vi "GeoData.vi"() -> ()   [LabVIEW 2017] (continued)
Altha\tFL\tCalhoun County\tH1\n32448\t12013\tMarianna\tFL\tCalhoun County\tH1\n32449\t12013\tWewahitchka\tFL\tCalhoun County\tH1\n32442\t12013\tGrand ridge\tFL\tCalhoun County\tH1\n34223\t12015\tEnglewood\tFL\tCharlotte County\tH1\n33950\t12015\tPunta gorda\tFL\tCharlotte County\tH1\n33947\t12015\tRotonda west\tFL\tCharlotte County\tH1\n33953\t12015\tPort charlotte\tFL\tCharlotte County\tH1\n34287\t12015\tNorth port\tFL\tCharlotte County\tH1\n33982\t12015\tPunta gorda\tFL\tCharlotte County\tH1\n34224\t12015\tEnglewood\tFL\tCharlotte County\tH1\n33938\t12015\tMurdock\tFL\tCharlotte County\tH1\n33949\t12015\tPort charlotte\tFL\tCharlotte County\tH1\n33983\t12015\tPunta gorda\tFL\tCharlotte County\tH1\n33952\t12015\tPort charlotte\tFL\tCharlotte County\tH1\n34266\t12015\tArcadia\tFL\tCharlotte County\tH1\n33981\t12015\tPort charlotte\tFL\tCharlotte County\tH1\n33980\t12015\tPunta gorda\tFL\tCharlotte County\tH1\n33946\t12015\tPlacida\tFL\tCharlotte County\tH1\n33954\t12015\tPort charlotte\tFL\tCharlotte County\tH1\n33955\t12015\tPunta gorda\tFL\tCharlotte County\tH1\n33951\t12015\tPunta gorda\tFL\tCharlotte County\tH1\n33917\t12015\tNorth fort myers\tFL\tCharlotte County\tH1\n33948\t12015\tPort charlotte\tFL\tCharlotte County\tH1\n34269\t12015\tArcadia\tFL\tCharlotte County\tH1\n34449\t12017\tInglis\tFL\tCitrus County\tH1\n34428\t12017\tCrystal river\tFL\tCitrus County\tH1\n34601\t12017\tBrooksville\tFL\tCitrus County\tH1\n34460\t12017\tLecanto\tFL\tCitrus County\tH1\n34464\t12017\tBeverly hills\tFL\tCitrus County\tH1\n34452\t12017\tInverness\tFL\tCitrus County\tH1\n34487\t12017\tHomosassa\tFL\tCitrus County\tH1\n34448\t12017\tHomosassa\tFL\tCitrus County\tH1\n34465\t12017\tBeverly hills\tFL\tCitrus County\tH1\n34434\t12017\tDunnellon\tFL\tCitrus County\tH1\n34450\t12017\tInverness\tFL\tCitrus County\tH1\n34436\t12017\tFloral city\tFL\tCitrus County\tH1\n34423\t12017\tCrystal river\tFL\tCitrus County\tH1\n34433\t12017\tDunnellon\tFL\tCitrus County\tH1\n34442\t12017\tHernando\tFL\tCitrus County\tH1\n34453\t12017\tInverness\tFL\tCitrus County\tH1\n34441\t12017\tHernando\tFL\tCitrus County\tH1\n34447\t12017\tHomosassa springs\tFL\tCitrus County\tH1\n34446\t12017\tHomosassa\tFL\tCitrus County\tH1\n34451\t12017\tInverness\tFL\tCitrus County\tH1\n34461\t12017\tLecanto\tFL\tCitrus County\tH1\n34445\t12017\tHolder\tFL\tCitrus County\tH1\n34429\t12017\tCrystal river\tFL\tCitrus County\tH1\n32050\t12019\tMiddleburg\tFL\tClay County\tH1\n32091\t12019\tStarke\tFL\tClay County\tH1\n32234\t12019\tJacksonville\tFL\tClay County\tH1\n32058\t12019\tLawtey\tFL\tClay County\tH1\n32656\t12019\tKeystone heights\tFL\tClay County\tH1\n32140\t12019\tFlorahome\tFL\tClay County\tH1\n32043\t12019\tGreen cove springs\tFL\tClay County\tH1\n32073\t12019\tOrange park\tFL\tClay County\tH1\n32666\t12019\tMelrose\tFL\tClay County\tH1\n32067\t12019\tOrange park\tFL\tClay County\tH1\n32079\t12019\tPenney farms\tFL\tClay County\tH1\n32160\t12019\tLake geneva\tFL\tClay County\tH1\n32003\t12019\tFleming island\tFL\tClay County\tH1\n32068\t12019\tMiddleburg\tFL\tClay County\tH1\n32006\t12019\tFleming island\tFL\tClay County\tH1\n32065\t12019\tOrange park\tFL\tClay County\tH1\n34119\t12021\tNaples\tFL\tCollier County\tH1\n34101\t12021\tNaples\tFL\tCollier County\tH1\n34112\t12021\tNaples\tFL\tCollier County\tH1\n34103\t12021\tNaples\tFL\tCollier County\tH1\n34114\t12021\tNaples\tFL\tCollier County\tH1\n34135\t12021\tBonita springs\tFL\tCollier County\tH1\n34141\t12021\tOchopee\tFL\tCollier County\tH1\n34146\t12021\tMarco island\tFL\tCollier County\tH1\n34110\t12021\tNaples\tFL\tCollier County\tH1\n34120\t12021\tNaples\tFL\tCollier County\tH1\n34134\t12021\tBonita springs\tFL\tCollier County\tH1\n34117\t12021\tNaples\tFL\tCollier County\tH1\n34106\t12021\tNaples\tFL\tCollier County\tH1\n34104\t12021\tNaples\tFL\tCollier County\tH1\n34116\t12021\tNaples\tFL\tCollier County\tH1\n34108\t12021\tNaples\tFL\tCollier County\tH1\n34145\t12021\tMarco island\tFL\tCollier County\tH1\n34140\t12021\tGoodland\tFL\tCollier County\tH1\n34102\t12021\tNaples\tFL\tCollier County\tH1\n34107\t12021\tNaples\tFL\tCollier County\tH1\n34109\t12021\tNaples\tFL\tCollier County\tH1\n34113\t12021\tNaples\tFL\tCollier County\tH1\n34105\t12021\tNaples\tFL\tCollier County\tH1\n34142\t12021\tImmokalee\tFL\tCollier County\tH1\n34139\t12021\tEverglades city\tFL\tCollier County\tH1\n34138\t12021\tChokoloskee\tFL\tCollier County\tH1\n32038\t12023\tFort white\tFL\tColumbia County\tH1\n32025\t12023\tLake city\tFL\tColumbia County\tH1\n32061\t12023\tLulu\tFL\tColumbia County\tH1\n32087\t12023\tSanderson\tFL\tColumbia County\tH1\n32096\t12023\tWhite springs\tFL\tColumbia County\tH1\n32056\t12023\tLake city\tFL\tColumbia County\tH1\n32643\t12023\tHigh springs\tFL\tColumbia County\tH1\n32024\t12023\tLake city\tFL\tColumbia County\tH1\n32055\t12023\tLake city\tFL\tColumbia County\tH1\n32094\t12023\tWellborn\tFL\tColumbia County\tH1\n34268\t12027\tNocatee\tFL\tDeSoto County\tH1\n34267\t12027\tFort ogden\tFL\tDeSoto County\tH1\n34266\t12027\tArcadia\tFL\tDeSoto County\tH1\n33865\t12027\tOna\tFL\tDeSoto County\tH1\n34269\t12027\tArcadia\tFL\tDeSoto County\tH1\n32008\t12029\tBranford\tFL\tDixie County\tH1\n32680\t12029\tOld town\tFL\tDixie County\tH1\n32692\t12029\tSuwannee\tFL\tDixie County\tH1\n32628\t12029\tCross city\tFL\tDixie County\tH1\n32648\t12029\tHorseshoe beach\tFL\tDixie County\tH1\n32359\t12029\tSteinhatchee\tFL\tDixie County\tH1\n32233\t12031\tAtlantic beach\tFL\tDuval County\tH6\n32244\t12031\tJacksonville\tFL\tDuval County\tH6\n32277\t12031\tJacksonville\tFL\tDuval County\tH6\n32209\t12031\tJacksonville\tFL\tDuval County\tH6\n32218\t12031\tJacksonville\tFL\tDuval County\tH6\n32250\t12031\tJacksonville beach\tFL\tDuval County\tH6\n32245\t12031\tJacksonville\tFL\tDuval County\tH6\n32212\t12031\tJacksonville\tFL\tDuval County\tH6\n32228\t12031\tJacksonville\tFL\tDuval County\tH6\n32229\t12031\tJacksonville\tFL\tDuval County\tH6\n32082\t12031\tPonte vedra beach\tFL\tDuval County\tH6\n32081\t12031\tPonte vedra\tFL\tDuval County\tH6\n32224\t12031\tJacksonville\tFL\tDuval County\tH6\n32234\t12031\tJacksonville\tFL\tDuval County\tH6\n32246\t12031\tJacksonville\tFL\tDuval County\tH6\n32214\t12031\tJacksonville\tFL\tDuval County\tH6\n32099\t12031\tJacksonville\tFL\tDuval County\tH6\n32084\t12031\tSaint augustine\tFL\tDuval County\tH6\n32221\t12031\tJacksonville\tFL\tDuval County\tH6\n32223\t12031\tJacksonville\tFL\tDuval County\tH6\n32219\t12031\tJacksonville\tFL\tDuval County\tH6\n32239\t12031\tJacksonville\tFL\tDuval County\tH6\n32227\t12031\tJacksonville\tFL\tDuval County\tH6\n32257\t12031\tJacksonville\tFL\tDuval County\tH6\n32073\t12031\tOrange park\tFL\tDuval County\tH6\n32205\t12031\tJacksonville\tFL\tDuval County\tH6\n32220\t12031\tJacksonville\tFL\tDuval County\tH6\n32226\t12031\tJacksonville\tFL\tDuval County\tH6\n32241\t12031\tJacksonville\tFL\tDuval County\tH6\n32208\t12031\tJacksonville\tFL\tDuval County\tH6\n32202\t12031\tJacksonville\tFL\tDuval County\tH6\n32211\t12031\tJacksonville\tFL\tDuval County\tH6\n32217\t12031\tJacksonville\tFL\tDuval County\tH6\n32222\t12031\tJacksonville\tFL\tDuval County\tH6\n32240\t12031\tJacksonville beach\tFL\tDuval County\tH6\n32254\t12031\tJacksonville\tFL\tDuval County\tH6\n32259\t12031\tSaint johns\tFL\tDuval County\tH6\n32235\t12031\tJacksonville\tFL\tDuval County\tH6\n32247\t12031\tJacksonville\tFL\tDuval County\tH6\n32206\t12031\tJacksonville\tFL\tDuval County\tH6\n32210\t12031\tJacksonville\tFL\tDuval County\tH6\n32216\t12031\tJacksonville\tFL\tDuval County\tH6\n32236\t12031\tJacksonville\tFL\tDuval County\tH6\n32256\t12031\tJacksonville\tFL\tDuval County\tH6\n32258\t12031\tJacksonville\tFL\tDuval County\tH6\n32255\t12031\tJacksonville\tFL\tDuval County\tH6\n32203\t12031\tJacksonville\tFL\tDuval County\tH6\n32204\t12031\tJacksonville\tFL\tDuval County\tH6\n32207\t12031\tJacksonville\tFL\tDuval County\tH6\n32225\t12031\tJacksonville\tFL\tDuval County\tH6\n32266\t12031\tNeptune beach\tFL\tDuval County\tH6\n32238\t12031\tJacksonville\tFL\tDuval County\tH6\n32506\t12033\tPensacola\tFL\tEscambia County\tH1\n32535\t12033\tCentury\tFL\tEscambia County\tH1\n32503\t12033\tPensacola\tFL\tEscambia County\tH1\n32520\t12033\tPensacola\tFL\tEscambia County\tH1\n32507\t12033\tPensacola\tFL\tEscambia County\tH1\n32524\t12033\tPensacola\tFL\tEscambia County\tH1\n32505\t12033\tPensacola\tFL\tEscambia County\tH1\n32568\t12033\tMc david\tFL\tEscambia County\tH1\n32511\t12033\tPensacola\tFL\tEscambia County\tH1\n32502\t12033\tPensacola\tFL\tEscambia County\tH1\n32534\t12033\tPensacola\tFL\tEscambia County\tH1\n32523\t12033\tPensacola\tFL\tEscambia County\tH1\n32577\t12033\tMolino\tFL\tEscambia County\tH1\n32560\t12033\tGonzalez\tFL\tEscambia County\tH1\n32509\t12033\tPensacola\tFL\tEscambia County\tH1\n32512\t12033\tPensacola\tFL\tEscambia County\tH1\n32504\t12033\tPensacola\tFL\tEscambia County\tH1\n32514\t12033\tPensacola\tFL\tEscambia County\tH1\n32526\t12033\tPensacola\tFL\tEscambia County\tH1\n32561\t12033\tGulf breeze\tFL\tEscambia County\tH1\n32513\t12033\tPensacola\tFL\tEscambia County\tH1\n32508\t12033\tPensacola\tFL\tEscambia County\tH1\n32516\t12033\tPensacola\tFL\tEscambia County\tH1\n32501\t12033\tPensacola\tFL\tEscambia County\tH1\n32522\t12033\tPensacola\tFL\tEscambia County\tH1\n32591\t12033\tPensacola\tFL\tEscambia County\tH1\n32533\t12033\tCantonment\tFL\tEscambia County\tH1\n32559\t12033\tPensacola\tFL\tEscambia County\tH1\n32145\t12035\tHastings\tFL\tFlagler County\tH1\n32143\t12035\tPalm coast\tFL\tFlagler County\tH1\n32110\t12035\tBunnell\tFL\tFlagler County\tH1\n32086\t12035\tSaint augustine\tFL\tFlagler County\tH1\n32136\t12035\tFlagler beach\tFL\tFlagler County\tH1\n32174\t12035\tOrmond beach\tFL\tFlagler County\tH1\n32164\t12035\tPalm coast\tFL\tFlagler County\tH1\n32135\t12035\tPalm coast\tFL\tFlagler County\tH1\n32080\t12035\tSaint augustine\tFL\tFlagler County\tH1\n32137\t12035\tPalm coast\tFL\tFlagler County\tH1\n32320\t12037\tApalachicola\tFL\tFranklin County\tH1\n32322\t12037\tCarrabelle\tFL\tFranklin County\tH1\n32358\t12037\tSopchoppy\tFL\tFranklin County\tH1\n32321\t12037\tBristol\tFL\tFranklin County\tH1\n32346\t12037\tPanacea\tFL\tFranklin County\tH1\n32328\t12037\tEastpoint\tFL\tFranklin County\tH1\n32324\t12039\tChattahoochee\tFL\tGadsden County\tH1\n32352\t12039\tQuincy\tFL\tGadsden County\tH1\n32332\t12039\tGretna\tFL\tGadsden County\tH1\n32343\t12039\tMidway\tFL\tGadsden County\tH1\n32330\t12039\tGreensboro\tFL\tGadsden County\tH1\n32351\t12039\tQuincy\tFL\tGadsden County\tH1\n32333\t12039\tHavana\tFL\tGadsden County\tH1\n32008\t12041\tBranford\tFL\tGilchrist County\tH1\n32669\t12041\tNewberry\tFL\tGilchrist County\tH1\n32619\t12041\tBell\tFL\tGilchrist County\tH1\n32693\t12041\tTrenton\tFL\tGilchrist County\tH1\n32643\t12041\tHigh springs\tFL\tGilchrist County\tH1\n33944\t12043\tPalmdale\tFL\tGlades County\tH1\n33471\t12043\tMoore haven\tFL\tGlades County\tH1\n34974\t12043\tOkeechobee\tFL\tGlades County\tH1\n33935\t12043\tLabelle\tFL\tGlades County\tH1\n33960\t12043\tVenus\tFL\tGlades County\tH1\n32456\t12045\tPort saint joe\tFL\tGulf County\tH1\n32465\t12045\tWewahitchka\tFL\tGulf County\tH1\n32052\t12047\tJasper\tFL\tHamilton County\tH1\n32053\t12047\tJennings\tFL\tHamilton County\tH1\n32096\t12047\tWhite springs\tFL\tHamilton County\tH1\n33841\t12049\tFort meade\tFL\tHardee County\tH1\n33873\t12049\tWauchula\tFL\tHardee County\tH1\n33890\t12049\tZolfo springs\tFL\tHardee County\tH1\n33834\t12049\tBowling green\tFL\tHardee County\tH1\n33865\t12049\tOna\tFL\tHardee County\tH1\n33975\t12051\tLabelle\tFL\tHendry County\tH1\n33471\t12051\tMoore haven\tFL\tHendry County\tH1\n33935\t12051\tLabelle\tFL\tHendry County\tH1\n33440\t12051\tClewiston\tFL\tHendry County\tH1\n33930\t12051\tFelda\tFL\tHendry County\tH1\n33936\t12051\tLehigh acres\tFL\tHendry County\tH1\n34142\t12051\tImmokalee\tFL\tHendry County\tH1\n34601\t12053\tBrooksville\tFL\tHernando County\tH1\n33523\t12053\tDade city\tFL\tHernando County\tH1\n33597\t12053\tWebster\tFL\tHernando County\tH1\n34613\t12053\tBrooksville\tFL\tHernando County\tH1\n34606\t12053\tSpring hill\tFL\tHernando County\tH1\n34608\t12053\tSpring hill\tFL\tHernando County\tH1\n34609\t12053\tSpring hill\tFL\tHernando County\tH1\n34607\t12053\tSpring hill\tFL\tHernando County\tH1\n34636\t12053\tIstachatta\tFL\tHernando County\tH1\n34604\t12053\tBrooksville\tFL\tHernando County\tH1\n34603\t12053\tBrooksville\tFL\tHernando County\tH1\n34602\t12053\tBrooksville\tFL\tHernando County\tH1\n34661\t12053\tNobleton\tFL\tHernando County\tH1\n34605\t12053\tBrooksville\tFL\tHernando County\tH1\n34614\t12053\tBrooksville\tFL\tHernando County\tH1\n34611\t12053\tSpring hill\tFL\tHernando County\tH1\n33843\t12055\tFrostproof\tFL\tHighlands County\tH1\n33875\t12055\tSebring\tFL\tHighlands County\tH1\n33862\t12055\tLake placid\tFL\tHighlands County\tH1\n33825\t12055\tAvon park\tFL\tHighlands County\tH1\n33876\t12055\tSebring\tFL\tHighlands County\tH1\n33871\t12055\tSebring\tFL\tHighlands County\tH1\n34974\t12055\tOkeechobee\tFL\tHighlands County\tH1\n33852\t12055\tLake placid\tFL\tHighlands County\tH1\n33870\t12055\tSebring\tFL\tHighlands County\tH1\n34266\t12055\tArcadia\tFL\tHighlands County\tH1\n33857\t12055\tLorida\tFL\tHighlands County\tH1\n33872\t12055\tSebring\tFL\tHighlands County\tH1\n33960\t12055\tVenus\tFL\tHighlands County\tH1\n33511\t12057\tBrandon\tFL\tHillsborough County\tH1\n33570\t12057\tRuskin\tFL\tHillsborough County\tH1\n33573\t12057\tSun city center\tFL\tHillsborough County\tH1\n33564\t12057\tPlant city\tFL\tHillsborough County\tH1\n33547\t12057\tLithia\tFL\tHillsborough County\tH1\n33583\t12057\tSeffner\tFL\tHillsborough County\tH1\n33614\t12057\tTampa\tFL\tHillsborough County\tH1\n33610\t12057\tTampa\tFL\tHillsborough County\tH1\n33616\t12057\tTampa\tFL\tHillsborough County\tH1\n33568\t12057\tRiverview\tFL\tHillsborough County\tH1\n33680\t12057\tTampa\tFL\tHillsborough County\tH1\n33694\t12057\tTampa\tFL\tHillsborough County\tH1\n33679\t12057\tTampa\tFL\tHillsborough County\tH1\n33565\t12057\tPlant city\tFL\tHillsborough County\tH1\n33544\t12057\tWesley chapel\tFL\tHillsborough County\tH1\n33605\t12057\tTampa\tFL\tHillsborough County\tH1\n33548\t12057\tLutz\tFL\tHillsborough County\tH1\n33617\t12057\tTampa\tFL\tHillsborough County\tH1\n33625\t12057\tTampa\tFL\tHillsborough County\tH1\n33615\t12057\tTampa\tFL\tHillsborough County\tH1\n33688\t12057\tTampa\tFL\tHillsborough County\tH1\n33558\t12057\tLutz\tFL\tHillsborough County\tH1\n33569\t12057\tRiverview\tFL\tHillsborough County\tH1\n33595\t12057\tValrico\tFL\tHillsborough County\tH1\n33611\t12057\tTampa\tFL\tHillsborough County\tH1\n33684\t12057\tTampa\tFL\tHillsborough County\tH1\n33620\t12057\tTampa\tFL\tHillsborough County\tH1\n33672\t12057\tTampa\tFL\tHillsborough County\tH1\n33646\t12057\tTampa\tFL\tHillsborough County\tH1\n33673\t12057\tTampa\tFL\tHillsborough County\tH1\n33630\t12057\tTampa\tFL\tHillsborough County\tH1\n33563\t12057\tPlant city\tFL\tHillsborough County\tH1\n33578\t12057\tRiverview\tFL\tHillsborough County\tH1\n33584\t12057\tSeffner\tFL\tHillsborough County\tH1\n33592\t12057\tThonotosassa\tFL\tHillsborough County\tH1\n33594\t12057\tValrico\tFL\tHillsborough County\tH1\n33623\t12057\tTampa\tFL\tHillsborough County\tH1\n33689\t12057\tTampa\tFL\tHillsborough County\tH1\n33674\t12057\tTampa\tFL\tHillsborough County\tH1\n33586\t12057\tSun city\tFL\tHillsborough County\tH1\n33549\t12057\tLutz\tFL\tHillsborough County\tH1\n33566\t12057\tPlant city\tFL\tHillsborough County\tH1\n33527\t12057\tDover\tFL\tHillsborough County\tH1\n33604\t12057\tTampa\tFL\tHillsborough County\tH1\n33598\t12057\tWimauma\tFL\tHillsborough County\tH1\n33624\t12057\tTampa\tFL\tHillsborough County\tH1\n33635\t12057\tTampa\tFL\tHillsborough County\tH1\n33687\t12057\tTampa\tFL\tHillsborough County\tH1\n33681\t12057\tTampa\tFL\tHillsborough County\tH1\n33559\t12057\tLutz\tFL\tHillsborough County\tH1\n33579\t12057\tRiverview\tFL\tHillsborough County\tH1\n33601\t12057\tTampa\tFL\tHillsborough County\tH1\n33602\t12057\tTampa\tFL\tHillsborough County\tH1\n33572\t12057\tApollo beach\tFL\tHillsborough County\tH1\n33550\t12057\tMango\tFL\tHillsborough County\tH1\n33596\t12057\tValrico\tFL\tHillsborough County\tH1\n33647\t12057\tTampa\tFL\tHillsborough County\tH1\n33626\t12057\tTampa\tFL\tHillsborough County\tH1\n33622\t12057\tTampa\tFL\tHillsborough County\tH1\n33609\t12057\tTampa\tFL\tHillsborough County\tH1\n33860\t12057\tMulberry\tFL\tHillsborough County\tH1\n33810\t12057\tLakeland\tFL\tHillsborough County\tH1\n33509\t12057\tBrandon\tFL\tHillsborough County\tH1\n33530\t12057\tDurant\tFL\tHillsborough County\tH1\n33675\t12057\tTampa\tFL\tHillsborough County\tH1\n33540\t12057\tZephyrhills\tFL\tHillsborough County\tH1\n33618\t12057\tTampa\tFL\tHillsborough County\tH1\n33629\t12057\tTampa\tFL\tHillsborough County\tH1\n33682\t12057\tTampa\tFL\tHillsborough County\tH1\n33621\t12057\tTampa\tFL\tHillsborough County\tH1\n33677\t12057\tTampa\tFL\tHillsborough County\tH1\n33571\t12057\tSun city center\tFL\tHillsborough County\tH1\n33503\t12057\tBalm\tFL\tHillsborough County\tH1\n33510\t12057\tBrandon\tFL\tHillsborough County\tH1\n33556\t12057\tOdessa\tFL\tHillsborough County\tH1\n33567\t12057\tPlant city\tFL\tHillsborough County\tH1\n33534\t12057\tGibsonton\tFL\tHillsborough County\tH1\n33606\t12057\tTampa\tFL\tHillsborough County\tH1\n33603\t12057\tTampa\tFL\tHillsborough County\tH1\n33613\t12057\tTampa\tFL\tHillsborough County\tH1\n33619\t12057\tTampa\tFL\tHillsborough County\tH1\n33634\t12057\tTampa\tFL\tHillsborough County\tH1\n33607\t12057\tTampa\tFL\tHillsborough County\tH1\n33612\t12057\tTampa\tFL\tHillsborough County\tH1\n33637\t12057\tTampa\tFL\tHillsborough County\tH1\n33685\t12057\tTampa\tFL\tHillsborough County\tH1\n33508\t12057\tBrandon\tFL\tHillsborough County\tH1\n33587\t12057\tSydney\tFL\tHillsborough County\tH1\n32455\t12059\tPonce de leon\tFL\tHolmes County\tH1\n32464\t12059\tWestville\tFL\tHolmes County\tH1\n32425\t12059\tBonifay\tFL\tHolmes County\tH1\n32433\t12059\tDefuniak springs\tFL\tHolmes County\tH1\n32440\t12059\tGraceville\tFL\tHolmes County\tH1\n32452\t12059\tNoma\tFL\tHolmes County\tH1\n32963\t12061\tVero beach\tFL\tIndian River County\tH1\n32965\t12061\tVero beach\tFL\tIndian River County\tH1\n32958\t12061\tSebastian\tFL\tIndian River County\tH1\n32966\t12061\tVero beach\tFL\tIndian River County\tH1\n32969\t12061\tVero beach\tFL\tIndian River County\tH1\n32960\t12061\tVero beach\tFL\tIndian River County\tH1\n32964\t12061\tVero beach\tFL\tIndian River County\tH1\n32957\t12061\tRoseland\tFL\tIndian River County\tH1\n32968\t12061\tVero beach\tFL\tIndian River County\tH1\n32961\t12061\tVero beach\tFL\tIndian River County\tH1\n32978\t12061\tSebastian\tFL\tIndian River County\tH1\n32948\t12061\tFellsmere\tFL\tIndian River County\tH1\n32967\t12061\tVero beach\tFL\tIndian River County\tH1\n32971\t12061\tWinter beach\tFL\tIndian River County\tH1\n32962\t12061\tVero beach\tFL\tIndian River County\tH1\n32970\t12061\tWabasso\tFL\tIndian River County\tH1\n32443\t12063\tGreenwood\tFL\tJackson County\tH1\n32428\t12063\tChipley\tFL\tJackson County\tH1\n32420\t12063\tAlford\tFL\tJackson County\tH1\n32438\t12063\tFountain\tFL\tJackson County\tH1\n32431\t12063\tCottondale\tFL\tJackson County\tH1\n32432\t12063\tCypress\tFL\tJackson County\tH1\n32423\t12063\tBascom\tFL\tJackson County\tH1\n32426\t12063\tCampbellton\tFL\tJackson County\tH1\n32445\t12063\tMalone\tFL\tJackson County\tH1\n32447\t12063\tMarianna\tFL\tJackson County\tH1\n32460\t12063\tSneads\tFL\tJackson County\tH1\n32440\t12063\tGraceville\tFL\tJackson County\tH1\n32446\t12063\tMarianna\tFL\tJackson County\tH1\n32448\t12063\tMarianna\tFL\tJackson County\tH1\n32442\t12063\tGrand ridge\tFL\tJackson County\tH1\n32309\t12065\tTallahassee\tFL\tJefferson County\tH1\n32331\t12065\tGreenville\tFL\tJefferson County\tH1\n32336\t12065\tLamont\tFL\tJefferson County\tH1\n32345\t12065\tMonticello\tFL\tJefferson County\tH1\n32361\t12065\tWacissa\tFL\tJefferson County\tH1\n32344\t12065\tMonticello\tFL\tJefferson County\tH1\n32337\t12065\tLloyd\tFL\tJefferson County\tH1\n32008\t12067\tBranford\tFL\tLafayette County\tH1\n32066\t12067\tMayo\tFL\tLafayette County\tH1\n32195\t12069\tWeirsdale\tFL\tLake County\tH1\n34731\t12069\tFruitland park\tFL\tLake County\tH1\n34729\t12069\tFerndale\tFL\tLake County\tH1\n32776\t12069\tSorrento\tFL\tLake County\tH1\n32784\t12069\tUmatilla\tFL\tLake County\tH1\n34797\t12069\tYalaha\tFL\tLake County\tH1\n32134\t12069\tFort mc coy\tFL\tLake County\tH1\n32163\t12069\tThe villages\tFL\tLake County\tH1\n32756\t12069\tMount dora\tFL\tLake County\tH1\n32767\t12069\tPaisley\tFL\tLake County\tH1\n34711\t12069\tClermont\tFL\tLake County\tH1\n34715\t12069\tClermont\tFL\tLake County\tH1\n34713\t12069\tClermont\tFL\tLake County\tH1\n32158\t12069\tLady lake\tFL\tLake County\tH1\n34756\t12069\tMontverde\tFL\tLake County\tH1\n32727\t12069\tEustis\tFL\tLake County\tH1\n32159\t12069\tLady lake\tFL\tLake County\tH1\n32757\t12069\tMount dora\tFL\tLake County\tH1\n34714\t12069\tClermont\tFL\tLake County\tH1\n34789\t12069\tLeesburg\tFL\tLake County\tH1\n34755\t12069\tMinneola\tFL\tLake County\tH1\n32102\t12069\tAstor\tFL\tLake County\tH1\n34712\t12069\tClermont\tFL\tLake County\tH1\n32702\t12069\tAltoona\tFL\tLake County\tH1\n32736\t12069\tEustis\tFL\tLake County\tH1\n34736\t12069\tGroveland\tFL\tLake County\tH1\n34748\t12069\tLeesburg\tFL\tLake County\tH1\n34762\t12069\tOkahumpka\tFL\tLake County\tH1\n34787\t12069\tWinter garden\tFL\tLake County\tH1\n34753\t12069\tMascotte\tFL\tLake County\tH1\n34705\t12069\tAstatula\tFL\tLake County\tH1\n34749\t12069\tLeesburg\tFL\tLake County\tH1\n32162\t12069\tThe villages\tFL\tLake County\tH1\n32720\t12069\tDeland\tFL\tLake County\tH1\n32726\t12069\tEustis\tFL\tLake County\tH1\n32778\t12069\tTavares\tFL\tLake County\tH1\n32735\t12069\tGrand island\tFL\tLake County\tH1\n34788\t12069\tLeesburg\tFL\tLake County\tH1\n34737\t12069\tHowey in the hills\tFL\tLake County\tH1\n33907\t12071\tFort myers\tFL\tLee County\tH1\n33908\t12071\tFort myers\tFL\tLee County\tH1\n33904\t12071\tCape coral\tFL\tLee County\tH1\n33916\t12071\tFort myers\tFL\tLee County\tH1\n33976\t12071\tLehigh acres\tFL\tLee County\tH1\n33922\t12071\tBokeelia\tFL\tLee County\tH1\n34119\t12071\tNaples\tFL\tLee County\tH1\n33991\t12071\tCape coral\tFL\tLee County\tH1\n33901\t12071\tFort myers\tFL\tLee County\tH1\n33971\t12071\tLehigh acres\tFL\tLee County\tH1\n33972\t12071\tLehigh acres\tFL\tLee County\tH1\n33956\t12071\tSaint james city\tFL\tLee County\tH1\n33990\t12071\tCape coral\tFL\tLee County\tH1\n34133\t12071\tBonita springs\tFL\tLee County\tH1\n33913\t12071\tFort myers\tFL\tLee County\tH1\n33914\t12071\tCape coral\tFL\tLee County\tH1\n33973\t12071\tLehigh acres\tFL\tLee County\tH1\n33919\t12071\tFort myers\tFL\tLee County\tH1\n33906\t12071\tFort myers\tFL\tLee County\tH1\n34135\t12071\tBonita springs\tFL\tLee County\tH1\n33903\t12071\tNorth fort myers\tFL\tLee County\tH1\n33902\t12071\tFort myers\tFL\tLee County\tH1\n33970\t12071\tLehigh acres\tFL\tLee County\tH1\n33965\t12071\tFort myers\tFL\tLee County\tH1\n33928\t12071\tEstero\tFL\tLee County\tH1\n33905\t12071\tFort myers\tFL\tLee County\tH1\n33915\t12071\tCape coral\tFL\tLee County\tH1\n34110\t12071\tNaples\tFL\tLee County\tH1\n34134\t12071\tBonita springs\tFL\tLee County\tH1\n33994\t12071\tFort myers\tFL\tLee County\tH1\n33924\t12071\tCaptiva\tFL\tLee County\tH1\n33912\t12071\tFort myers\tFL\tLee County\tH1\n33957\t12071\tSanibel\tFL\tLee County\tH1\n33974\t12071\tLehigh acres\tFL\tLee County\tH1\n33993\t12071\tCape coral\tFL\tLee County\tH1\n33918\t12071\tNorth fort myers\tFL\tLee County\tH1\n33910\t12071\tCape coral\tFL\tLee County\tH1\n33945\t12071\tPineland\tFL\tLee County\tH1\n33921\t12071\tBoca grande\tFL\tLee County\tH1\n33920\t12071\tAlva\tFL\tLee County\tH1\n33967\t12071\tFort myers\tFL\tLee County\tH1\n33966\t12071\tFort myers\tFL\tLee County\tH1\n33955\t12071\tPunta gorda\tFL\tLee County\tH1\n34136\t12071\tBonita springs\tFL\tLee County\tH1\n33917\t12071\tNorth fort myers\tFL\tLee County\tH1\n33936\t12071\tLehigh acres\tFL\tLee County\tH1\n33909\t12071\tCape coral\tFL\tLee County\tH1\n33931\t12071\tFort myers beach\tFL\tLee County\tH1\n33932\t12071\tFort myers beach\tFL\tLee County\tH1\n33929\t12071\tEstero\tFL\tLee County\tH1\n33911\t12071\tFort myers\tFL\tLee County\tH1\n32305\t12073\tTallahassee\tFL\tLeon County\tH1\n32315\t12073\tTallahassee\tFL\tLeon County\tH1\n32399\t12073\tTallahassee\tFL\tLeon County\tH1\n32314\t12073\tTallahassee\tFL\tLeon County\tH1\n32302\t12073\tTallahassee\tFL\tLeon County\tH1\n32313\t12073\tTallahassee\tFL\tLeon County\tH1\n32304\t12073\tTallahassee\tFL\tLeon County\tH1\n32309\t12073\tTallahassee\tFL\tLeon County\tH1\n32327\t12073\tCrawfordville\tFL\tLeon County\tH1\n32311\t12073\tTallahassee\tFL\tLeon County\tH1\n32318\t12073\tTallahassee\tFL\tLeon County\tH1\n32303\t12073\tTallahassee\tFL\tLeon County\tH1\n32308\t12073\tTallahassee\tFL\tLeon County\tH1\n32310\t12073\tTallahassee\tFL\tLeon County\tH1\n32312\t12073\tTallahassee\tFL\tLeon County\tH1\n32362\t12073\tWoodville\tFL\tLeon County\tH1\n32301\t12073\tTallahassee\tFL\tLeon County\tH1\n32317\t12073\tTallahassee\tFL\tLeon County\tH1\n32306\t12073\tTallahassee\tFL\tLeon County\tH1\n32307\t12073\tTallahassee\tFL\tLeon County\tH1\n32395\t12073\tTallahassee\tFL\tLeon County\tH1\n32316\t12073\tTallahassee\tFL\tLeon County\tH1\n34449\t12075\tInglis\tFL\tLevy County\tH1\n32626\t12075\tChiefland\tFL\tLevy County\tH1\n32621\t12075\tBronson\tFL\tLevy County\tH1\n32669\t12075\tNewberry\tFL\tLevy County\tH1\n32693\t12075\tTrenton\tFL\tLevy County\tH1\n32683\t12075\tOtter creek\tFL\tLevy County\tH1\n32618\t12075\tArcher\tFL\tLevy County\tH1\n32696\t12075\tWilliston\tFL\tLevy County\tH1\n32639\t12075\tGulf hammock\tFL\tLevy County\tH1\n32625\t12075\tCedar key\tFL\tLevy County\tH1\n34498\t12075\tYankeetown\tFL\tLevy County\tH1\n32668\t12075\tMorriston\tFL\tLevy County\tH1\n34431\t12075\tDunnellon\tFL\tLevy County\tH1\n32644\t12075\tChiefland\tFL\tLevy County\tH1\n32334\t12077\tHosford\tFL\tLiberty County\tH1\n32321\t12077\tBristol\tFL\tLiberty County\tH1\n32351\t12077\tQuincy\tFL\tLiberty County\tH1\n32360\t12077\tTelogia\tFL\tLiberty County\tH1\n32350\t12079\tPinetta\tFL\tMadison County\tH1\n32331\t12079\tGreenville\tFL\tMadison County\tH1\n32336\t12079\tLamont\tFL\tMadison County\tH1\n32059\t12079\tLee\tFL\tMadison County\tH1\n32340\t12079\tMadison\tFL\tMadison County\tH1\n34208\t12081\tBradenton\tFL\tManatee County\tH1\n34264\t12081\tOneco\tFL\tManatee County\tH1\n34270\t12081\tTallevast\tFL\tManatee County\tH1\n34206\t12081\tBradenton\tFL\tManatee County\tH1\n34221\t12081\tPalmetto\tFL\tManatee County\tH1\n34209\t12081\tBradenton\tFL\tManatee County\tH1\n34217\t12081\tBradenton beach\tFL\tManatee County\tH1\n34222\t12081\tEllenton\tFL\tManatee County\tH1\n34251\t12081\tMyakka city\tFL\tManatee County\tH1\n34243\t12081\tSarasota\tFL\tManatee County\tH1\n34205\t12081\tBradenton\tFL\tManatee County\tH1\n34280\t12081\tBradenton\tFL\tManatee County\tH1\n34216\t12081\tAnna maria\tFL\tManatee County\tH1\n34282\t12081\tBradenton\tFL\tManatee County\tH1\n34228\t12081\tLongboat key\tFL\tManatee County\tH1\n34202\t12081\tBradenton\tFL\tManatee County\tH1\n34211\t12081\tBradenton\tFL\tManatee County\tH1\n34240\t12081\tSarasota\tFL\tManatee County\tH1\n34212\t12081\tBradenton\tFL\tManatee County\tH1\n34201\t12081\tBradenton\tFL\tManatee County\tH1\n33598\t12081\tWimauma\tFL\tManatee County\tH1\n34266\t12081\tArcadia\tFL\tManatee County\tH1\n34220\t12081\tPalmetto\tFL\tManatee County\tH1\n33834\t12081\tBowling green\tFL\tManatee County\tH1\n34210\t12081\tBradenton\tFL\tManatee County\tH1\n34219\t12081\tParrish\tFL\tManatee County\tH1\n34203\t12081\tBradenton\tFL\tManatee County\tH1\n34204\t12081\tBradenton\tFL\tManatee County\tH1\n34260\t12081\tSarasota\tFL\tManatee County\tH1\n34250\t12081\tTerra ceia\tFL\tManatee County\tH1\n34207\t12081\tBradenton\tFL\tManatee County\tH1\n34215\t12081\tCortez\tFL\tManatee County\tH1\n32195\t12083\tWeirsdale\tFL\tMarion County\tH1\n32182\t12083\tOrange springs\tFL\tMarion County\tH1\n34471\t12083\tOcala\tFL\tMarion County\tH1\n34480\t12083\tOcala\tFL\tMarion County\tH1\n34482\t12083\tOcala\tFL\tMarion County\tH1\n32784\t12083\tUmatilla\tFL\tMarion County\tH1\n32664\t12083\tMc intosh\tFL\tMarion County\tH1\n34430\t12083\tDunnellon\tFL\tMarion County\tH1\n32663\t12083\tLowell\tFL\tMarion County\tH1\n32111\t12083\tCandler\tFL\tMarion County\tH1\n34491\t12083\tSummerfield\tFL\tMarion County\tH1\n34475\t12083\tOcala\tFL\tMarion County\tH1\n34481\t12083\tOcala\tFL\tMarion County\tH1\n32134\t12083\tFort mc coy\tFL\tMarion County\tH1\n32113\t12083\tCitra\tFL\tMarion County\tH1\n32667\t12083\tMicanopy\tFL\tMarion County\tH1\n34473\t12083\tOcala\tFL\tMarion County\tH1\n34474\t12083\tOcala\tFL\tMarion County\tH1\n32634\t12083\tFairfield\tFL\tMarion County\tH1\n34472\t12083\tOcala\tFL\tMarion County\tH1\n34476\t12083\tOcala\tFL\tMarion County\tH1\n32192\t12083\tSparr\tFL\tMarion County\tH1\n32681\t12083\tOrange lake\tFL\tMarion County\tH1\n32133\t12083\tEastlake weir\tFL\tMarion County\tH1\n32696\t12083\tWilliston\tFL\tMarion County\tH1\n34420\t12083\tBelleview\tFL\tMarion County\tH1\n34477\t12083\tOcala\tFL\tMarion County\tH1\n34492\t12083\tSummerfield\tFL\tMarion County\tH1\n34483\t12083\tOcala\tFL\tMarion County\tH1\n32686\t12083\tReddick\tFL\tMarion County\tH1\n34470\t12083\tOcala\tFL\tMarion County\tH1\n32702\t12083\tAltoona\tFL\tMarion County\tH1\n32617\t12083\tAnthony\tFL\tMarion County\tH1\n32668\t12083\tMorriston\tFL\tMarion County\tH1\n34431\t12083\tDunnellon\tFL\tMarion County\tH1\n34432\t12083\tDunnellon\tFL\tMarion County\tH1\n34484\t12083\tOxford\tFL\tMarion County\tH1\n34488\t12083\tSilver springs\tFL\tMarion County\tH1\n34478\t12083\tOcala\tFL\tMarion County\tH1\n34479\t12083\tOcala\tFL\tMarion County\tH1\n32162\t12083\tThe villages\tFL\tMarion County\tH1\n32179\t12083\tOcklawaha\tFL\tMarion County\tH1\n34489\t12083\tSilver springs\tFL\tMarion County\tH1\n33478\t12085\tJupiter\tFL\tMartin County\tH1\n34994\t12085\tStuart\tFL\tMartin County\tH1\n34956\t12085\tIndiantown\tFL\tMartin County\tH1\n34995\t12085\tStuart\tFL\tMartin County\tH1\n34974\t12085\tOkeechobee\tFL\tMartin County\tH1\n34957\t12085\tJensen beach\tFL\tMartin County\tH1\n34996\t12085\tStuart\tFL\tMartin County\tH1\n34958\t12085\tJensen beach\tFL\tMartin County\tH1\n34992\t12085\tPort salerno\tFL\tMartin County\tH1\n33438\t12085\tCanal point\tFL\tMartin County\tH1\n33458\t12085\tJupiter\tFL\tMartin County\tH1\n33475\t12085\tHobe sound\tFL\tMartin County\tH1\n33455\t12085\tHobe sound\tFL\tMartin County\tH1\n34990\t12085\tPalm city\tFL\tMartin County\tH1\n34991\t12085\tPalm city\tFL\tMartin County\tH1\n33469\t12085\tJupiter\tFL\tMartin County\tH1\n34997\t12085\tStuart\tFL\tMartin County\tH1\n33015\t12086\tHialeah\tFL\tMiami-Dade County\tH1\n33137\t12086\tMiami\tFL\tMiami-Dade County\tH1\n33176\t12086\tMiami\tFL\tMiami-Dade County\tH1\n33166\t12086\tMiami\tFL\tMiami-Dade County\tH1\n33283\t12086\tMiami\tFL\tMiami-Dade County\tH1\n33030\t12086\tHomestead\tFL\tMiami-Dade County\tH1\n33114\t12086\tCoral gables\tFL\tMiami-Dade County\tH1\n33116\t12086\tMiami\tFL\tMiami-Dade County\tH1\n33002\t12086\tHialeah\tFL\tMiami-Dade County\tH1\n33192\t12086\tMiami\tFL\tMiami-Dade County\tH1\n33199\t12086\tMiami\tFL\tMiami-Dade County\tH1\n33129\t12086\tMiami\tFL\tMiami-Dade County\tH1\n33109\t12086\tMiami beach\tFL\tMiami-Dade County\tH1\n33127\t12086\tMiami\tFL\tMiami-Dade County\tH1\n33145\t12086\tMiami\tFL\tMiami-Dade County\tH1\n33175\t12086\tMiami\tFL\tMiami-Dade County\tH1\n33189\t12086\tMiami\tFL\tMiami-Dade County\tH1\n33245\t12086\tMiami\tFL\tMiami-Dade County\tH1\n33011\t12086\tHialeah\tFL\tMiami-Dade County\tH1\n33017\t12086\tHialeah\tFL\tMiami-Dade County\tH1\n33269\t12086\tMiami\tFL\tMiami-Dade County\tH1\n33247\t12086\tMiami\tFL\tMiami-Dade County\tH1\n33195\t12086\tMiami\tFL\tMiami-Dade County\tH1\n33198\t12086\tMiami\tFL\tMiami-Dade County\tH1\n33206\t12086\tMiami\tFL\tMiami-Dade County\tH1\n33014\t12086\tHialeah\tFL\tMiami-Dade County\tH1\n33016\t12086\tHialeah\tFL\tMiami-Dade County\tH1\n33012\t12086\tHialeah\tFL\tMiami-Dade County\tH1\n33130\t12086\tMiami\tFL\tMiami-Dade County\tH1\n33135\t12086\tMiami\tFL\tMiami-Dade County\tH1\n33126\t12086\tMiami\tFL\tMiami-Dade County\tH1\n33134\t12086\tMiami\tFL\tMiami-Dade County\tH1\n33144\t12086\tMiami\tFL\tMiami-Dade County\tH1\n33146\t12086\tMiami\tFL\tMiami-Dade County\tH1\n33149\t12086\tKey biscayne\tFL\tMiami-Dade County\tH1\n33169\t12086\tMiami\tFL\tMiami-Dade County\tH1\n33154\t12086\tMiami beach\tFL\tMiami-Dade County\tH1\n33183\t12086\tMiami\tFL\tMiami-Dade County\tH1\n33027\t12086\tHollywood\tFL\tMiami-Dade County\tH1\n33056\t12086\tMiami gardens\tFL\tMiami-Dade County\tH1\n33031\t12086\tHomestead\tFL\tMiami-Dade County\tH1\n33234\t12086\tMiami\tFL\tMiami-Dade County\tH1\n33266\t12086\tMiami\tFL\tMiami-Dade County\tH1\n33013\t12086\tHialeah\tFL\tMiami-Dade County\tH1\n33023\t12086\tHollywood\tFL\tMiami-Dade County\tH1\n33133\t12086\tMiami\tFL\tMiami-Dade County\tH1\n33141\t12086\tMiami beach\tFL\tMiami-Dade County\tH1\n33168\t12086\tMiami\tFL\tMiami-Dade County\tH1\n33172\t12086\tMiami\tFL\tMiami-Dade County\tH1\n33174\t12086\tMiami\tFL\tMiami-Dade County\tH1\n33167\t12086\tMiami\tFL\tMiami-Dade County\tH1\n33181\t12086\tMiami\tFL\tMiami-Dade County\tH1\n33184\t12086\tMiami\tFL\tMiami-Dade County\tH1\n33190\t12086\tMiami\tFL\tMiami-Dade County\tH1\n33055\t12086\tOpa locka\tFL\tMiami-Dade County\tH1\n33034\t12086\tHomestead\tFL\tMiami-Dade County\tH1\n33261\t12086\tMiami\tFL\tMiami-Dade County\tH1\n33231\t12086\tMiami\tFL\tMiami-Dade County\tH1\n33197\t12086\tMiami\tFL\tMiami-Dade County\tH1\n33106\t12086\tMiami\tFL\tMiami-Dade County\tH1\n33139\t12086\tMiami beach\tFL\tMiami-Dade County\tH1\n33142\t12086\tMiami\tFL\tMiami-Dade County\tH1\n33140\t12086\tMiami beach\tFL\tMiami-Dade County\tH1\n33150\t12086\tMiami\tFL\tMiami-Dade County\tH1\n33101\t12086\tMiami\tFL\tMiami-Dade County\tH1\n33160\t12086\tNorth miami beach\tFL\tMiami-Dade County\tH1\n33170\t12086\tMiami\tFL\tMiami-Dade County\tH1\n33179\t12086\tMiami\tFL\tMiami-Dade County\tH1\n33177\t12086\tMiami\tFL\tMiami-Dade County\tH1\n33196\t12086\tMiami\tFL\tMiami-Dade County\tH1\n33185\t12086\tMiami\tFL\tMiami-Dade County\tH1\n33193\t12086\tMiami\tFL\tMiami-Dade County\tH1\n33242\t12086\tMiami\tFL\tMiami-Dade County\tH1\n33194\t12086\tMiami\tFL\tMiami-Dade County\tH1\n33032\t12086\tHomestead\tFL\tMiami-Dade County\tH1\n33033\t12086\tHomestead\tFL\tMiami-Dade County\tH1\n33152\t12086\tMiami\tFL\tMiami-Dade County\tH1\n33280\t12086\tMiami\tFL\tMiami-Dade County\tH1\n33164\t12086\tMiami\tFL\tMiami-Dade County\tH1\n33153\t12086\tMiami\tFL\tMiami-Dade County\tH1\n33191\t12086\tMiami\tFL\tMiami-Dade County\tH1\n33018\t12086\tHialeah\tFL\tMiami-Dade County\tH1\n33131\t12086\tMiami\tFL\tMiami-Dade County\tH1\n33161\t12086\tMiami\tFL\tMiami-Dade County\tH1\n33173\t12086\tMiami\tFL\tMiami-Dade County\tH1\n33157\t12086\tMiami\tFL\tMiami-Dade County\tH1\n33182\t12086\tMiami\tFL\tMiami-Dade County\tH1\n33239\t12086\tMiami beach\tFL\tMiami-Dade County\tH1\n33128\t12086\tMiami\tFL\tMiami-Dade County\tH1\n33243\t12086\tMiami\tFL\tMiami-Dade County\tH1\n33238\t12086\tMiami\tFL\tMiami-Dade County\tH1\n33010\t12086\tHialeah\tFL\tMiami-Dade County\tH1\n33138\t12086\tMiami\tFL\tMiami-Dade County\tH1\n33122\t12086\tMiami\tFL\tMiami-Dade County\tH1\n33125\t12086\tMiami\tFL\tMiami-Dade County\tH1\n33147\t12086\tMiami\tFL\tMiami-Dade County\tH1\n33090\t12086\tHomestead\tFL\tMiami-Dade County\tH1\n33178\t12086\tMiami\tFL\tMiami-Dade County\tH1\n33255\t12086\tMiami\tFL\tMiami-Dade County\tH1\n33296\t12086\tMiami\tFL\tMiami-Dade County\tH1\n33186\t12086\tMiami\tFL\tMiami-Dade County\tH1\n33257\t12086\tMiami\tFL\tMiami-Dade County\tH1\n33187\t12086\tMiami\tFL\tMiami-Dade County\tH1\n33035\t12086\tHomestead\tFL\tMiami-Dade County\tH1\n33092\t12086\tHomestead\tFL\tMiami-Dade County\tH1\n33124\t12086\tMiami\tFL\tMiami-Dade County\tH1\n33119\t12086\tMiami beach\tFL\tMiami-Dade County\tH1\n33136\t12086\tMiami\tFL\tMiami-Dade County\tH1\n33143\t12086\tMiami\tFL\tMiami-Dade County\tH1\n33132\t12086\tMiami\tFL\tMiami-Dade County\tH1\n33162\t12086\tMiami\tFL\tMiami-Dade County\tH1\n33165\t12086\tMiami\tFL\tMiami-Dade County\tH1\n33156\t12086\tMiami\tFL\tMiami-Dade County\tH1\n33155\t12086\tMiami\tFL\tMiami-Dade County\tH1\n33158\t12086\tMiami\tFL\tMiami-Dade County\tH1\n33180\t12086\tMiami\tFL\tMiami-Dade County\tH1\n33256\t12086\tMiami\tFL\tMiami-Dade County\tH1\n33265\t12086\tMiami\tFL\tMiami-Dade County\tH1\n33054\t12086\tOpa locka\tFL\tMiami-Dade County\tH1\n33222\t12086\tMiami\tFL\tMiami-Dade County\tH1\n33233\t12086\tMiami\tFL\tMiami-Dade County\tH1\n33163\t12086\tMiami\tFL\tMiami-Dade County\tH1\n33112\t12086\tMiami\tFL\tMiami-Dade County\tH1\n33039\t12086\tHomestead\tFL\tMiami-Dade County\tH1\n33040\t12087\tKey west\tFL\tMonroe County\tH1\n33043\t12087\tBig pine key\tFL\tMonroe County\tH1\n33070\t12087\tTavernier\tFL\tMonroe County\tH1\n33036\t12087\tIslamorada\tFL\tMonroe County\tH1\n33045\t12087\tKey west\tFL\tMonroe County\tH1\n33001\t12087\tLong key\tFL\tMonroe County\tH1\n33034\t12087\tHomestead\tFL\tMonroe County\tH1\n33052\t12087\tMarathon shores\tFL\tMonroe County\tH1\n33050\t12087\tMarathon\tFL\tMonroe County\tH1\n33042\t12087\tSummerland key\tFL\tMonroe County\tH1\n33041\t12087\tKey west\tFL\tMonroe County\tH1\n33051\t12087\tKey colony beach\tFL\tMonroe County\tH1\n33037\t12087\tKey largo\tFL\tMonroe County\tH1\n32046\t12089\tHilliard\tFL\tNassau County\tH1\n32234\t12089\tJacksonville\tFL\tNassau County\tH1\n32011\t12089\tCallahan\tFL\tNassau County\tH1\n32035\t12089\tFernandina beach\tFL\tNassau County\tH1\n32041\t12089\tYulee\tFL\tNassau County\tH1\n32009\t12089\tBryceville\tFL\tNassau County\tH1\n32034\t12089\tFernandina beach\tFL\tNassau County\tH1\n32097\t12089\tYulee\tFL\tNassau County\tH1\n32547\t12091\tFort walton beach\tFL\tOkaloosa County\tH1\n32539\t12091\tCrestview\tFL\tOkaloosa County\tH1\n32578\t12091\tNiceville\tFL\tOkaloosa County\tH1\n32580\t12091\tValparaiso\tFL\tOkaloosa County\tH1\n32549\t12091\tFort walton beach\tFL\tOkaloosa County\tH1\n32541\t12091\tDestin\tFL\tOkaloosa County\tH1\n32540\t12091\tDestin\tFL\tOkaloosa County\tH1\n32588\t12091\tNiceville\tFL\tOkaloosa County\tH1\n32536\t12091\tCrestview\tFL\tOkaloosa County\tH1\n32542\t12091\tEglin afb\tFL\tOkaloosa County\tH1\n32564\t12091\tHolt\tFL\tOkaloosa County\tH1\n32579\t12091\tShalimar\tFL\tOkaloosa County\tH1\n32548\t12091\tFort walton beach\tFL\tOkaloosa County\tH1\n32569\t12091\tMary esther\tFL\tOkaloosa County\tH1\n32531\t12091\tBaker\tFL\tOkaloosa County\tH1\n32544\t12091\tHurlburt field\tFL\tOkaloosa County\tH1\n32567\t12091\tLaurel hill\tFL\tOkaloosa County\tH1\n34972\t12093\tOkeechobee\tFL\tOkeechobee County\tH1\n34974\t12093\tOkeechobee\tFL\tOkeechobee County\tH1\n34973\t12093\tOkeechobee\tFL\tOkeechobee County\tH1\n32710\t12095\tClarcona\tFL\tOrange County\tH1\n32824\t12095\tOrlando\tFL\tOrange County\tH1\n32828\t12095\tOrlando\tFL\tOrange County\tH1\n32798\t12095\tZellwood\tFL\tOrange County\tH1\n34747\t12095\tKissimmee\tFL\tOrange County\tH1\n32793\t12095\tWinter park\tFL\tOrange County\tH1\n32804\t12095\tOrlando\tFL\tOrange County\tH1\n32835\t12095\tOrlando\tFL\tOrange County\tH1\n32858\t12095\tOrlando\tFL\tOrange County\tH1\n32877\t12095\tOrlando\tFL\tOrange County\tH1\n32830\t12095\tOrlando\tFL\tOrange County\tH1\n32765\t12095\tOviedo\tFL\tOrange County\tH1\n32776\t12095\tSorrento\tFL\tOrange County\tH1\n32777\t12095\tTangerine\tFL\tOrange County\tH1\n34777\t12095\tWinter garden\tFL\tOrange County\tH1\n32861\t12095\tOrlando\tFL\tOrange County\tH1\n34760\t12095\tOakland\tFL\tOrange County\tH1\n32867\t12095\tOrlando\tFL\tOrange County\tH1\n32817\t12095\tOrlando\tFL\tOrange County\tH1\n32832\t12095\tOrlando\t
